vi "report-test-started.vi"(8 "error in (no error)":errorcluster) -> (0 "error out":errorcluster)   [LabVIEW 2019]
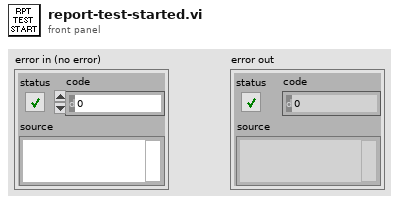
[diagram p1: front panel]
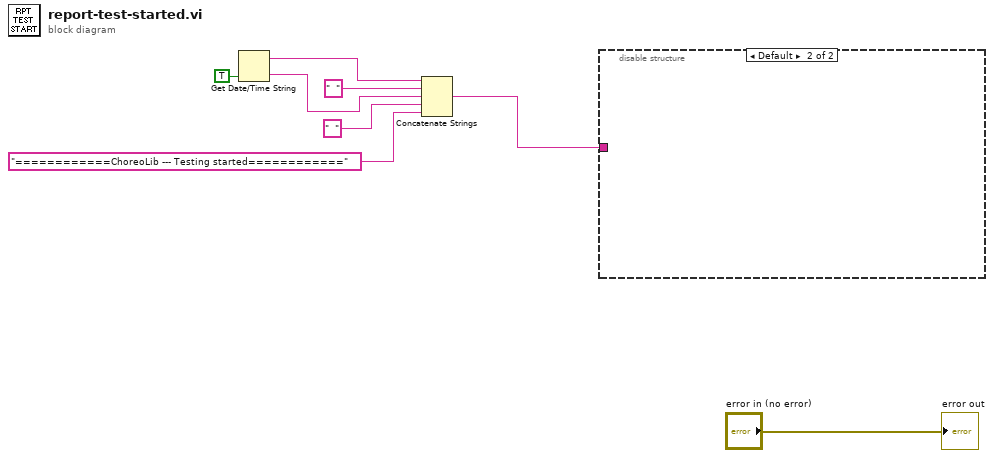
[diagram p0: block diagram]
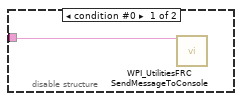
[diagram p2: hidden frame]
diagram:
  n1 = Get Date/Time String(want seconds? (F)=TRUE) -> (date string=w6:string, time string=w4:string)  [unwired: 2 in]
  n2 = Concatenate Strings(w6, "  " ("string"), w4, "  " ("string"), "============ChoreoLib --- Testing started============" ("string")) -> (w1:string)
  n3 = disable-structure shown="Default" {
    disable-tunnel: w1 -> [w9 _]
    frame condition #0 {
      n4 = call <vilib>:"WPI_UtilitiesFRC SendMessageToConsole.vi"("Message"=w9) -> ()  [unwired: 14 in, 1 out]
    }
    frame condition #1 (active) {
    }
  }
  "error out" <- "error in (no error)"
